vi "Serrure numérique V2 1.vi"() -> ()   [LabVIEW 2018]
uses:
  Global 1.vi
panel:
  out "Max":dbl
  out "Tentive":dbl
  in  "OK Button":bool
  out "Rouge":bool
  out "Vert":bool
  in  "N°3":i8(knob) scale=1.0..9.0
  in  "N°2":i8(knob) scale=1.0..9.0
  in  "N°1":i8(knob) scale=0.0..9.0
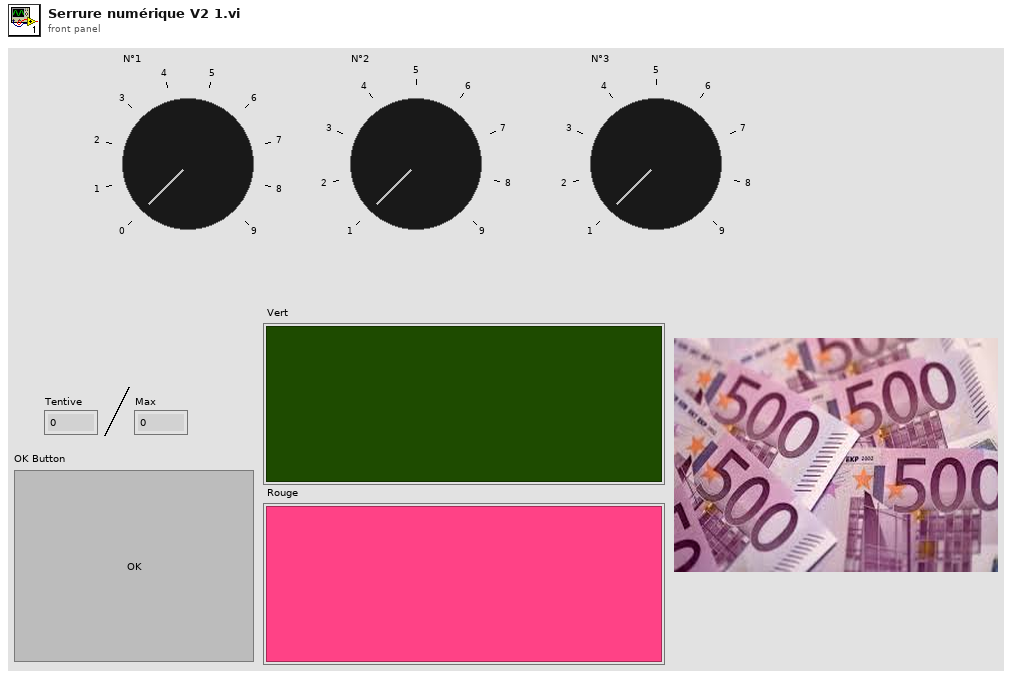
[diagram p1: front panel]
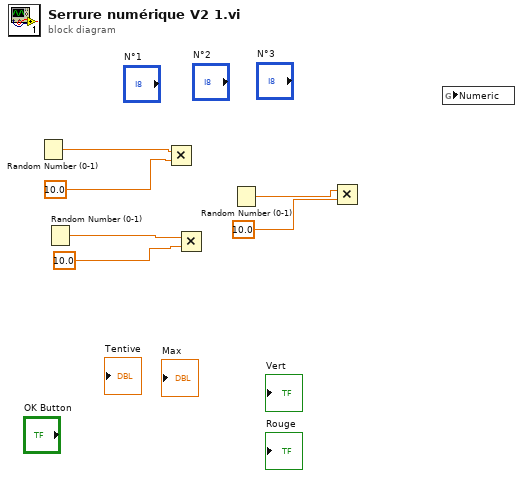
[diagram p0: block diagram]
diagram:
  n1 = Random Number (0-1)() -> (number: 0 to 1=w6:dbl)
  n2 = Random Number (0-1)() -> (number: 0 to 1=w4:dbl)
  n3 = Multiply(x=w6, y=10.0) -> ()  [unwired: 1 out]
  n4 = Multiply(x=w4, y=10.0) -> ()  [unwired: 1 out]
  n5 = Random Number (0-1)() -> (number: 0 to 1=w2:dbl)
  n6 = Multiply(x=w2, y=10.0) -> ()  [unwired: 1 out]
  n7 = global read "Global 1.vi" "Numeric"() -> ()  [unwired: 1 in]
